vi "DAQ_Host.vi"() -> ()   [LabVIEW 2017]
uses:
  <vilib>/Utility/file.llb/Read Delimited Spreadsheet (string).vi
  <vilib>/Utility/file.llb/Write Delimited Spreadsheet (string).vi
  <vilib>/Utility/file.llb/Write Delimited Spreadsheet (DBL).vi
  <resource>/objmgr/ni.dex.rc
panel:
  in  "Error In":errorcluster
  out "Number of Disconnections":u32
  out "Available Elements for Reading":i32
  out "DAQ?":bool
  in  "Stop DAQ":bool
  out "Error Out":errorcluster
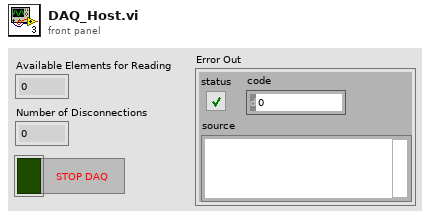
[diagram p1: front panel]
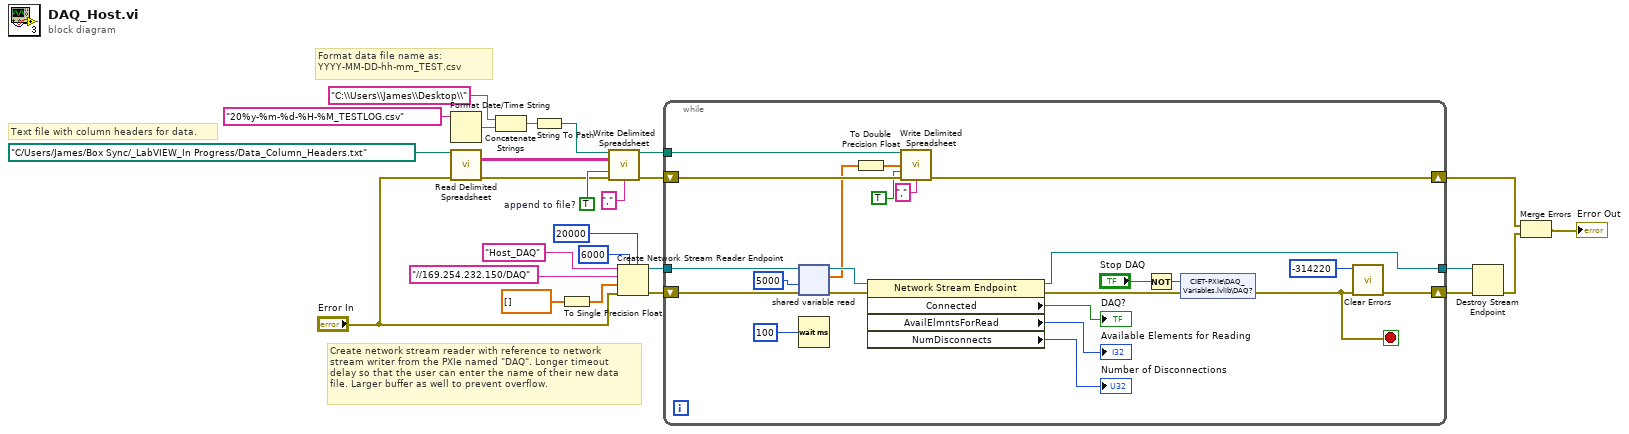
[diagram p0: block diagram]
diagram:
  w13 = TRUE  # append to file?
  # "Format data file name as:\nYYYY-MM-DD-hh-mm_TEST.csv"
  # "Create network stream reader with reference to network\nstream writer from the PXIe named \"DAQ\". Longer timeout\ndelay so that the user can enter the name of their new data\nfile. Larger buffer as well to prevent overflow."
  # "Text file with column headers for data."
  n1 = Format Date/Time String(time format string (%c)="20%y-%m-%d-%H-%M_TESTLOG.csv") -> (date/time string=w3:string)  [unwired: 2 in]
  n2 = call-poly <vilib>:"Read Delimited Spreadsheet.vi"("file path (dialog if empty)"=path "C:/Users/James/Box Sync/_LabVIEW_In Progress/Data_Column_Headers.txt", "error in (no error)"="Error In") -> ("all rows"=w16:string[][], "error out"=w11:errorcluster)  [unwired: 8 in, 4 out]
  n3 = Concatenate Strings("C:\\Users\\James\\Desktop\\" ("string"), w3) -> (w5:string)
  n4 = String To Path(string=w5) -> (path=w2:path)
  n5 = To Single Precision Float(number=dbl[] []) -> (single precision float=w24:sgl[])
  n6 = call-poly <vilib>:"Write Delimited Spreadsheet.vi"("file path (dialog if empty)"=w2, "2D data"=w16, "append to file? (new file:F)"=w13, "error in (no error)"=w11, "delimiter (\\t)"=",") -> ("new file path (Not A Path if cancelled)"=w12:path, "error out"=w10:errorcluster)  [unwired: 9 in]
  n7 = Create Network Stream Reader Endpoint(5:20000 ("timeout in ms (-1)"), 7:6000 ("reader buffer size"), 8:"Error In", 9:w24, 10:"//169.254.232.150/DAQ" ("writer url"), 11:"Host_DAQ" ("reader name")) -> (0:w21:errorcluster, 3:w20:refnum<k21>)  [unwired: 1 in]
  n8 = while {
    shift-right: [w38] -> w19
    shift-left: w21 -> [w46]
    tunnel: w20 -> [w47]
    tunnel: [w37] -> w18
    tunnel: w12 -> [w33]
    shift-right: [w31] -> w9
    shift-left: w10 -> [w32]
    stop <- w36 stop-if-true
    n9 = shared-variable-read(w47, w46, 5000 ("timeout ms (-1)")) -> (w43:refnum<k21>, w41:errorcluster, w30:sgl[])  [unwired: 1 out]
    n10 = Wait (ms)(milliseconds to wait=u32 100) -> ()  [unwired: 1 out]
    n11 = To Double Precision Float(number=w30) -> (double precision float=w27:dbl[])
    n12 = property class="Network Stream Endpoint"(reference=w43, error in=w41) -> (reference out=w37:refnum<k21>, error out=w42:errorcluster, "Connected"=→"DAQ?":bool, "AvailElmntsForRead"=→"Available Elements for Reading":i32, "NumDisconnects"=→"Number of Disconnections":u32)
    n13 = call-poly <vilib>:"Write Delimited Spreadsheet.vi"("file path (dialog if empty)"=w33, "1D data"=w27, "append to file? (new file:F)"=TRUE, "error in (no error)"=w32, "delimiter (\\t)"="," ("delimiter (\\t)")) -> ("error out"=w31:errorcluster)  [unwired: 9 in, 1 out]
    n14 = Not(x="Stop DAQ") -> (.not. x?=w45:bool)
    n15 = shared-variable "CIET-PXIe\\DAQ_Variables.lvlib\\DAQ?"(w45, error in=w42) -> (error out=w36:errorcluster)
    n16 = call <vilib>:"Clear Errors.vi"("error in (no error)"=w36, "specific error code to clear (0: all)"=-314220) -> ("error out"=w38:errorcluster)  [unwired: 4 in, 1 out]
  }
  n17 = Destroy Stream Endpoint(8:w19, 11:w18) -> (0:w8:errorcluster)
  n18 = Merge Errors(w9, w8) -> (→"Error Out":errorcluster)
